vi "Read Errors.vi"(0 "FPGA API in":refnum<class "FPGA API Concrete.lvclass">, 11 "error in (no error)":errorcluster) -> (4 "FPGA API out":refnum<class "FPGA API Concrete.lvclass">, 8 "Errors":errorcluster[](array[cluster]), 15 "error out":errorcluster)   [LabVIEW 2019, in "FPGA API Concrete.lvclass"]
uses:
  FPGA API Concrete.lvclass
  FPGA API Concrete.lvclass/FPGA API Concrete.ctl
  <vilib>/Utility/error.llb/Error Cluster From Error Code.vi
  <vilib>/rvi/errors/niLvFpgaAdjustHostInterfaceError.vi
  <vilib>/rvi/interface/nirviReadWriteControl/nirviReadWriteControl.xnode
  FPGA Ref.ctl
  NiFpgaLv.dll
  <vilib>/rvi/interface/Simulation/niFpgaSimulationCallBeginRW.vi
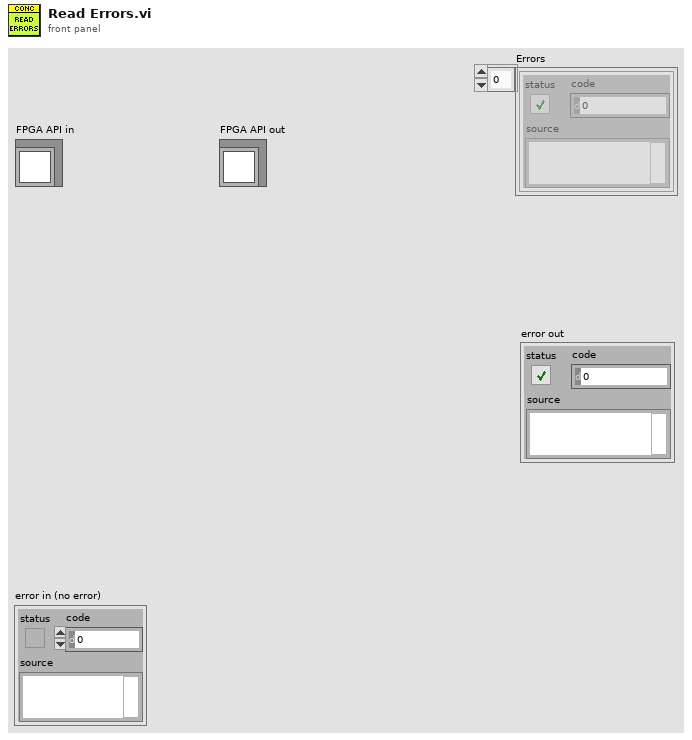
[diagram p1: front panel]
types:
  T1 = typedef "FPGA API Concrete.lvclass/FPGA Ref.ctl" = refnum<k20>
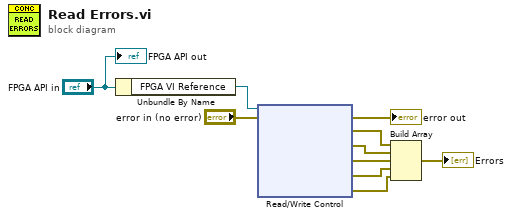
[diagram p0: block diagram]
diagram:
  n1 = Unbundle By Name("FPGA API in") -> ("FPGA VI Reference"=w8:T1)
  n2 = xnode "Read/Write Control"("FPGA VI Reference In"=w8, "error in"="error in (no error)") -> ("error out"=→"error out":errorcluster, "Error DI"=w6:errorcluster, "Error DO"=w5:errorcluster, "Error AI mod 1"=w4:errorcluster, "Error AI mod 2"=w3:errorcluster, "Error AO"=w2:errorcluster)  [unwired: 1 out]
  n3 = Build Array(w6, w5, w4, w3, w2) -> (→"Errors":errorcluster[])
  "FPGA API out" <- "FPGA API in"
